vi "UV-VIS SetPreAmpGain.vi"(3 "error in (no error)":errorcluster, 4 "index":i32, 5 "Control in":refnum<class "CCD_camera.lvclass">) -> (0 "error out":errorcluster, 1 "DLL error code":u32, 2 "Control out":refnum<class "CCD_camera.lvclass">)   [LabVIEW 2020, in "CCD_camera.lvclass"]
doc: "This function will set the pre amp gain to be used for subsequent acquisitions. The actual gain factor that will be applied can be found through a call to the <B>GetPreAmpGain</B> function. The number of Pre Amp Gains available is found by calling the <B>GetNumberPreAmpGains</B> function. \n\n<B>Parameter:</B>\nindex - gain required\n Valid values: 0 to <B>GetNumberPreAmpGains</B>-1\n\n<B>Error codes:</B>\nDRV_SUCCESS - Pre amp gain set.\nDRV_NOT_INITIALIZED - System not initialized.\nDRV_ACQUIRING - Acquisition in progress.\nDRV_P1INVALID - Index out of range."
uses:
  CCD_camera.lvclass
  C:/dev/TRANCON/Classes/Detector/Detector.lvclass
  Detector.lvclass/Detector.ctl
  Detector.lvclass
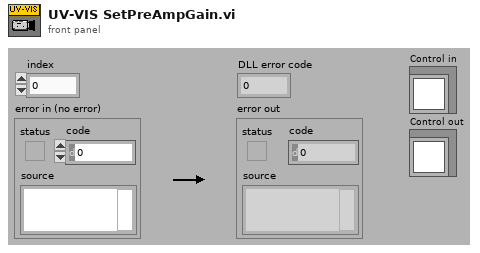
[diagram p1: front panel]
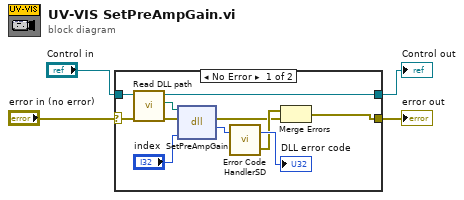
[diagram p0: block diagram]
diagram:
  n1 = case shown="No Error" "error in (no error)" {
    selector: "error in (no error)" -> [w11 w17]
    tunnel: [w6 w17] -> w3
    tunnel: [w5 w16] -> w2
    tunnel: "Control in" -> [w12 w16]
    frame No Error {
      n2 = call "Read DLL path.vi"("error in (no error)"=w11, "Detector in"=w12) -> ("error out"=w9:errorcluster, "DLL path"=w10:path, "Detector out"=w5:refnum<class "CCD_camera.lvclass">)  [unwired: 7 in]
      n3 = dll-call lib="S:/TRANCON/DLL/Atmcd32d.dll" fn="SetPreAmpGain"(path in=w10, error in=w9, "index"="index") -> (error out=w7:errorcluster, "return type"=w15:u32)  [unwired: 2 in, 1 out]
      n4 = call "Error Code HandlerSD.vi"("DLL error code"=w15) -> ("error out"=w8:errorcluster, "dup DLL error code"=→"DLL error code":u32)  [unwired: 1 in]
      n5 = Merge Errors(w8, w7) -> (w6:errorcluster)
    }
    frame Error {
    }
  }
  "error out" <- w3
  "Control out" <- w2
